vi "Práctica01_Ejercicio2_1.vi"() -> ()   [LabVIEW 2020]
panel:
  in  "stop":bool
  out "Meter":dbl(knob) scale=0.0..100.0
  in  "Knob":dbl(knob) scale=0.0..100.0
  out "Boolean 2":bool
  in  "Boolean":bool
  out "Mensaje impreso":string
  in  "Inserte mensaje":string
  out "Age":u8(slide) scale=0.0..100.0
  in  "Edad":dbl
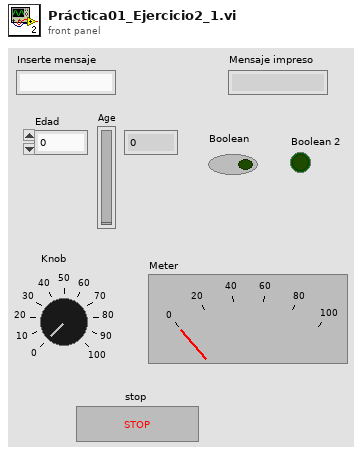
[diagram p1: front panel]
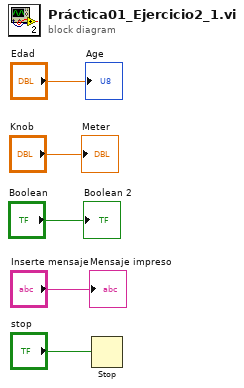
[diagram p0: block diagram]
diagram:
  n1 = Stop(stop? (T)="stop") -> ()
  "Age" <- "Edad"
  "Mensaje impreso" <- "Inserte mensaje"
  "Boolean 2" <- "Boolean"
  "Meter" <- "Knob"
